vi "configuration UI.vi"() -> ()   [LabVIEW 2013, in "Shared Library Module editor node.lvclass"]
doc: "Platypus Framework 1.0.1.60\nNI Systems Engineering - National Instruments"
uses:
  Shared Library Module editor node.lvclass
  <vilib>/NI/Configuration Framework/Node/NodeRef.ctl
  <vilib>/NI/Configuration Framework/Node/NISE_CEF_Node.lvclass
  <vilib>/NI/AMC/Message Queue.ctl
  <vilib>/NI/AMC/Message.ctl
  <vilib>/NI/Tools/Keyed Array/KeyedArray.ctl
  <vilib>/NI/Configuration Framework/Node/UserEventRef.ctl
  <vilib>/NI/Configuration Framework/Controls/EventCluster.ctl
  <vilib>/NI/DCAF UI Toolkit/Controls/Configure.ctl
  <vilib>/NI/DCAF UI Toolkit/Controls/Add.ctl
  <vilib>/NI/DCAF UI Toolkit/Controls/Remove.ctl
  <vilib>/NI/DCAF UI Toolkit/Controls/Import.ctl
  configuration/Shared Library Module configuration.lvclass
  <vilib>/Utility/miscctls.llb/LVPositionTypeDef.ctl
  <vilib>/NI/Module Execution Interface/Engine Configuration/engine configuration.lvclass
  <vilib>/NI/Tag Bus Data Framework/Configuration Editor/Classes/Engine Parent/Engine Parent Editor Node.lvclass
  <vilib>/NI/Configuration Framework/serializable configuration/NISE_CEF_serializable configuration.lvclass/NISE_CEF_serializable configuration.ctl
  configuration/Shared Library Module configuration.lvclass/Shared Library Module configuration.ctl
  <vilib>/NI/Tag Bus/tag/tag descriptor.lvclass/tag descriptor.ctl
  <vilib>/NI/Tag Bus/tag/write tag name.vi
  configuration/Write args.vi
  configuration/Write dllpath.vi
  Write local path.vi
  Read local path.vi
  <vilib>/NI/Configuration Framework/serializable configuration/Read UID.vi
  configuration/Read args.vi
  configuration/Read dllpath.vi
  <vilib>/NI/Tag Bus Data Framework/Configuration Editor/Classes/Module editor node/Read Module Configuration.vi
  <vilib>/NI/Configuration Framework/serializable configuration/read metadata property.vi
  <vilib>/NI/Tag Bus Data Framework/Configuration Editor/Classes/Module editor node/Write Module Configuration.vi
  <vilib>/Utility/LVClass/Get LV Class Name.vi
  <vilib>/NI/Configuration Framework/error generator/NISE_error generator.vi
  <vilib>/NI/Configuration Framework/serializable configuration/set metadata property.vi
  <vilib>/NI/Configuration Framework/serializable configuration/NISE_CEF_serializable configuration.lvclass
  <vilib>/NI/Tag Bus Module Framework/module configuration/TBM module configuration.lvclass
  <vilib>/NI/Configuration Framework/NISE_CEF_TreeControl.lvlib
  <vilib>/NI/Tag Bus Data Framework/Configuration Editor/Classes/Module editor node/module editor node.lvclass
  <vilib>/NI/Tag Bus Module Framework/channel/TBM channel.lvclass
  <vilib>/NI/Tools/Keyed Array/Tools_KeyedArray.lvlib
  <vilib>/NI/AMC/AMC.lvlib
  <vilib>/NI/DCAF UI Toolkit/Controls/DCAF UI Elements.lvlib
panel:
  in  "Top Level Tab Control":T1(tab)
  in  "Open Button":T2
  in  "settings":T3
  in  "channel":i32(listbox)
  in  "Add Button":T4
  in  "Remove Button":T5
  in  "Additional Arguments":string[](array[string])
  in  "Library Path (required)":path
  in  "Local Library Path (optional)":path
  in  "user event":T6
  in  "main queue":T7
  in  "node ref":T8
  # "It is recommended that libraries are placed in the default search path. For example, on Linux RT this would be /usr/lib, while VxWorks places it at /ni-rt/system.\n\nIf this is the case, libraries can be referenced by name. To make the name cross-platform, wildcards can be specified.\n\nLibname.* becomes libname.dll on windows and libname.so on Linux.\n\nLibname*.* becomes Libname32.* on 32-bit operating systems/environments and Libname64.* on 64-bit operating systems/environments."
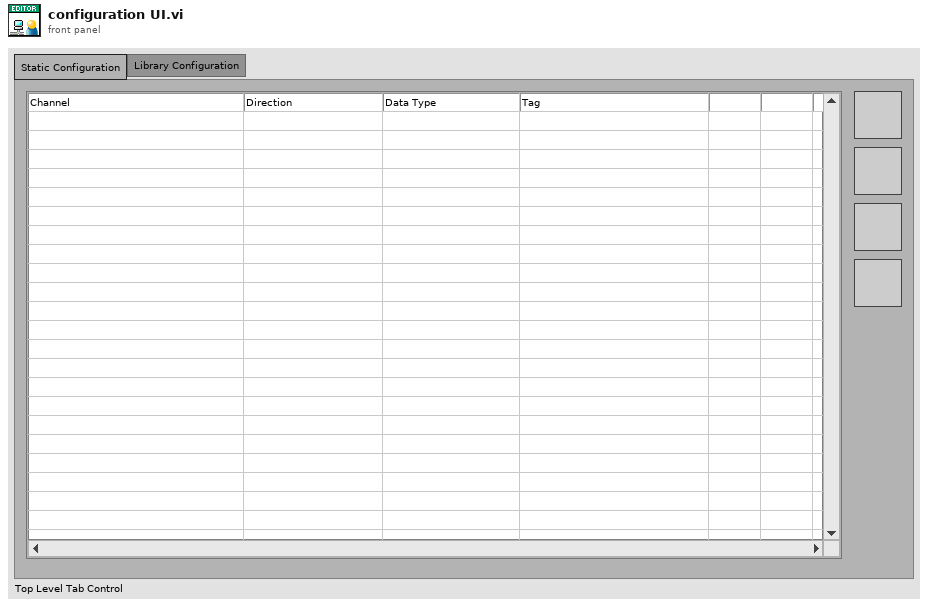
[diagram p1: front panel]
types:
  T1 = enum32{"Static Configuration", "Library Configuration"}
  T2 = typedef "DCAF UI Elements.lvlib/Import.ctl" = bool
  T3 = typedef "DCAF UI Elements.lvlib/Configure.ctl" = bool
  T4 = typedef "DCAF UI Elements.lvlib/Add.ctl" = bool
  T5 = typedef "DCAF UI Elements.lvlib/Remove.ctl" = bool
  T6 = typedef "NISE_CEF_Node.lvclass/UserEventRef.ctl" = refnum<user-event>
  T7 = typedef "AMC.lvlib/Message Queue.ctl" = refnum<queue>
  T8 = typedef "NISE_CEF_Node.lvclass/NodeRef.ctl" = refnum<data-value>
  T9 = typedef "LVPositionTypeDef.ctl" = cluster{"Left":i32, "Top":i32}
  T10 = typedef "NISE_CEF_TreeControl.lvlib/EventCluster.ctl" = cluster{"command":string, "data":string}
  T11 = typedef "Shared Library Module editor node.lvclass/table line.ctl" = cluster{"channel in":refnum<class "TBM channel.lvclass">, "tag name":string}
  T12 = typedef "TBM channel.lvclass/channel classification.ctl" = enum16{"input data", "output data", "processing parameter", "processing result"}
  T13 = typedef "tag bus.lvlib/tag descriptor.lvclass/Data Type.ctl" = enum16{"Double", "Single", "I64", "I32", "I16", "I8", "U64", "U32", "U16", "U8", "Boolean", "String", "Array of Double", "Array of Single", "Array of I64", "Array of I32", "Array of I16", "Array of I8", "Array of U64", "Array of U32", "Array of U16", "Array of U8", "Array of Boolean", "Array of String"}
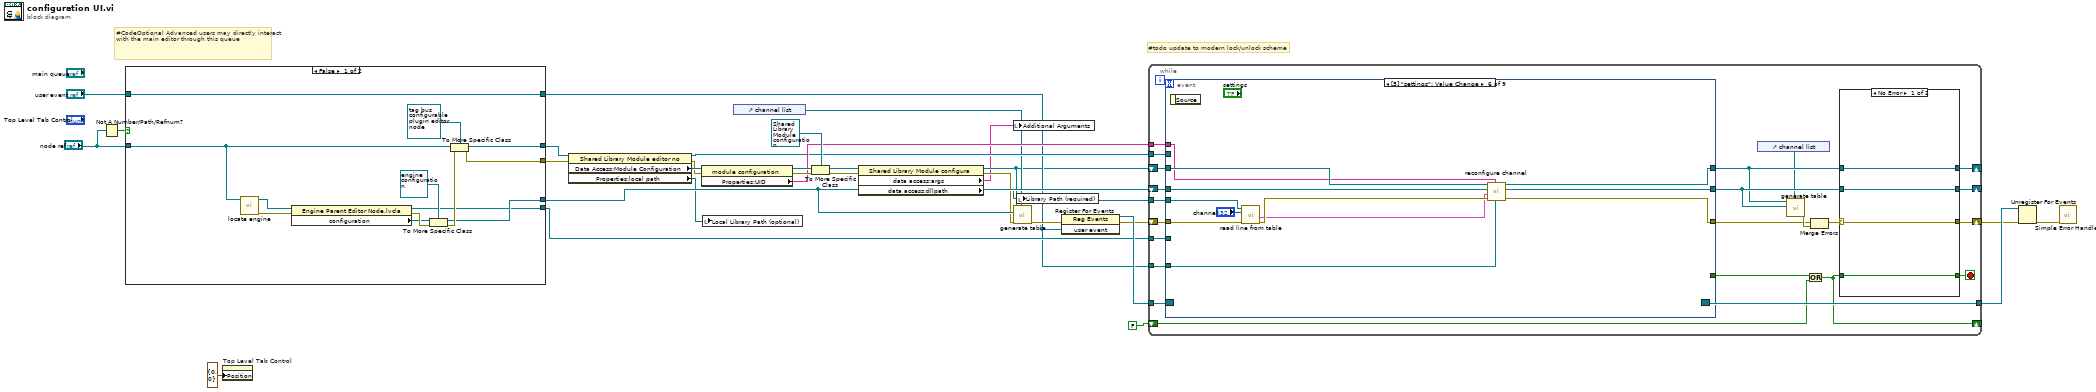
[diagram p0: block diagram]
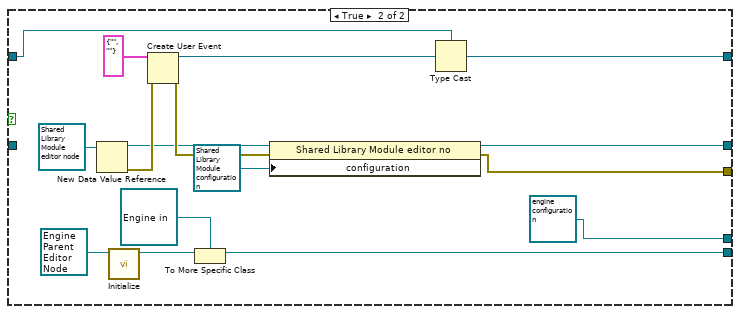
[diagram p2: hidden frame]
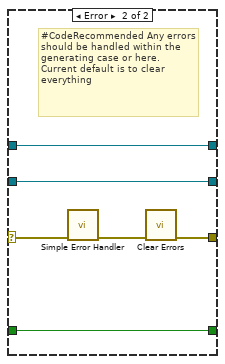
[diagram p3: hidden frame]
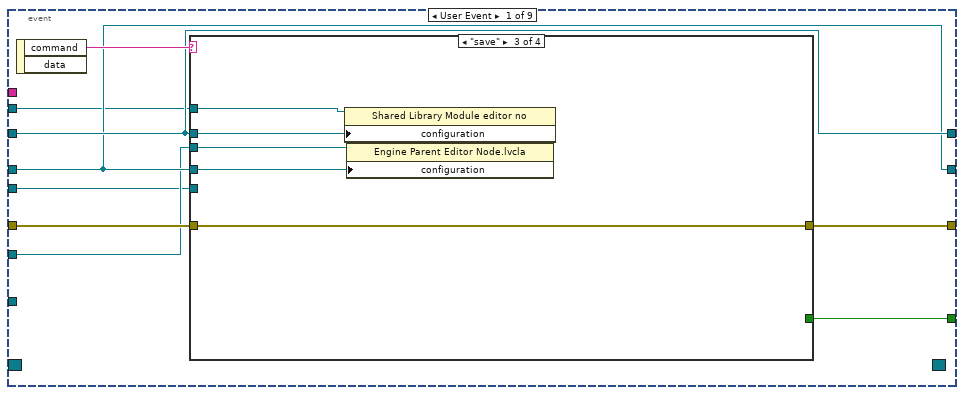
[diagram p4: hidden frame]
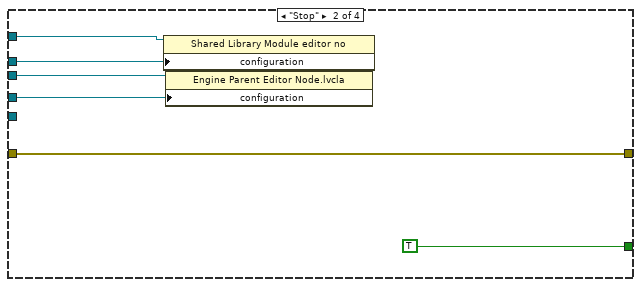
[diagram p6: hidden frame]
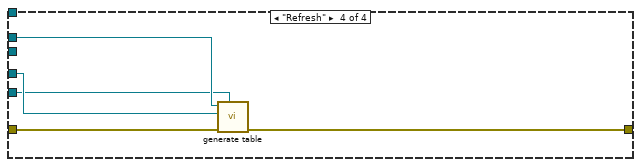
[diagram p7: hidden frame]
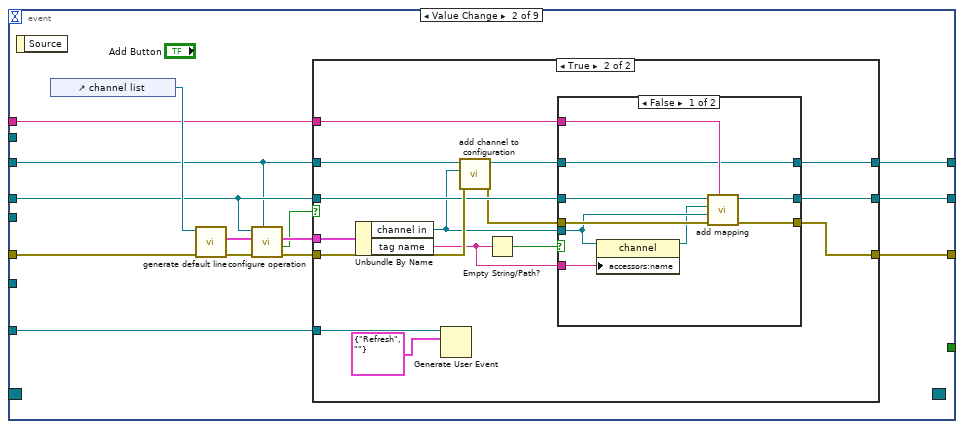
[diagram p8: hidden frame]
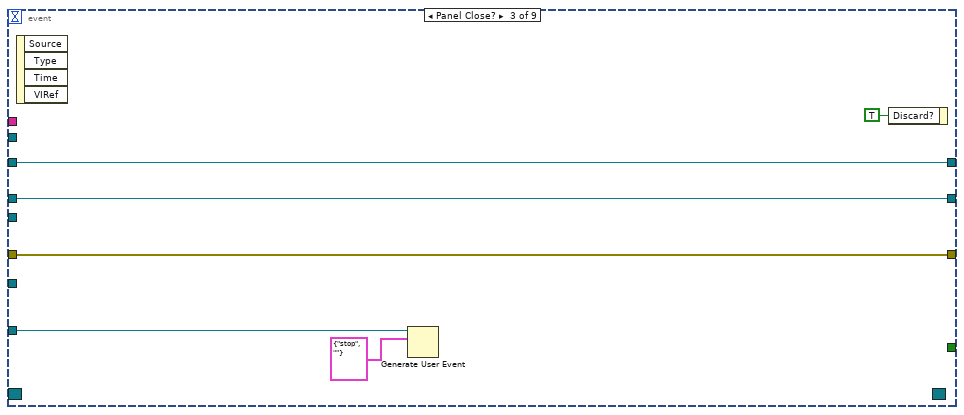
[diagram p11: hidden frame]
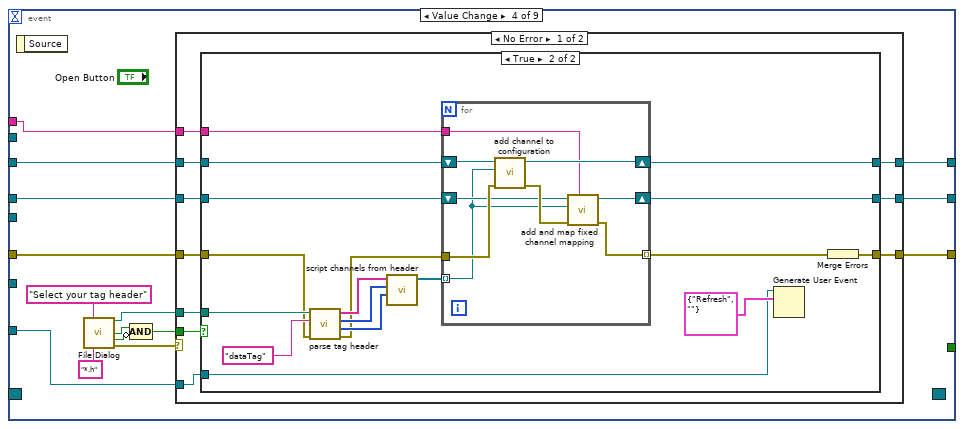
[diagram p12: hidden frame]
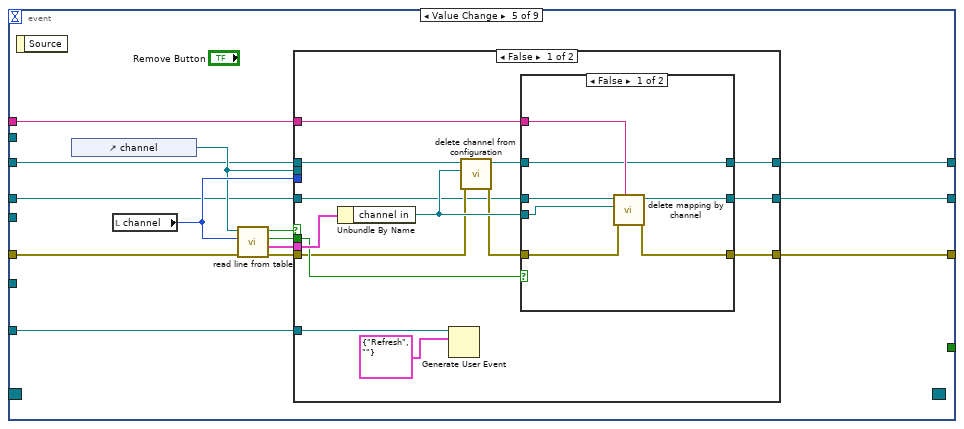
[diagram p15: hidden frame]
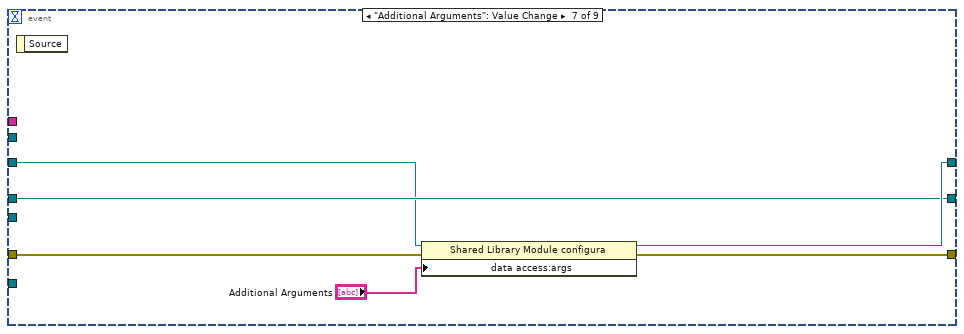
[diagram p18: hidden frame]
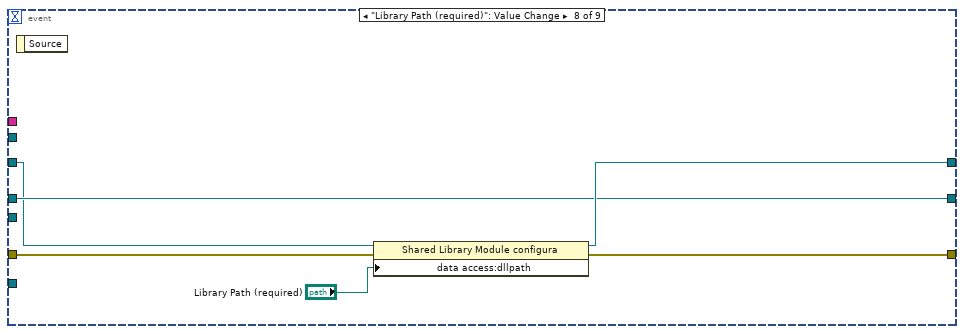
[diagram p19: hidden frame]
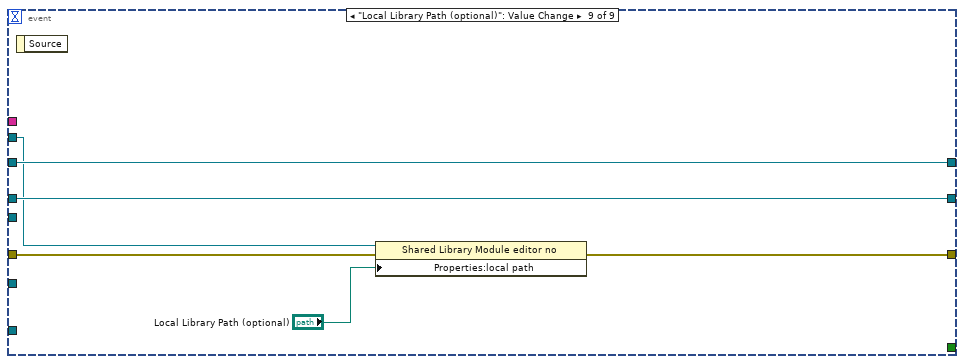
[diagram p20: hidden frame]
diagram:
  # "#todo update to modern lock/unlock scheme"
  # "#CodeOptional Advanced users may directly interact with the main editor through this queue"
  n1 = Not A Number/Path/Refnum?(number/path/refnum="node ref") -> (NaN/Path/Refnum?=w22:bool)
  n2 = case shown="False" w22 {
    tunnel: "user event" -> [w44 w46]
    tunnel: [w44 w47] -> w8
    tunnel: "node ref" -> [w42 _]
    tunnel: [w41 w54] -> w15
    tunnel: [w40 w48] -> w20
    tunnel: [w33 refnum<class "engine configuration.lvclass"> refnum ("Engine Configuration")] -> w17
    tunnel: [w32 w51] -> w11
    frame False {
      n3 = call <vilib>:"locate engine.vi"("component"=w42) -> ("error out"=w37:errorcluster, "engine"=w39:refnum<data-value>)  [unwired: 9 in]
      n4 = property class="Engine Parent Editor Node.lvcla"(reference=w39, error in=w37) -> (reference out=w32:refnum<data-value>, error out=w36:errorcluster, "configuration"=w35:refnum<class "NISE_CEF_serializable configuration.lvclass">)
      n5 = To More Specific Class(target class=refnum<class "engine configuration.lvclass"> refnum ("engine configuration.lvclass"), reference=w35, error in=w36) -> (specific class reference=w33:refnum<class "engine configuration.lvclass">, error out=w34:errorcluster)
      n6 = To More Specific Class(target class=refnum<data-value> refnum ("data value reference"), reference=w42, error in=w34) -> (specific class reference=w41:refnum<data-value>, error out=w40:errorcluster)
    }
    frame True {
      n7 = New Data Value Reference(data value=refnum<class "Shared Library Module editor node.lvclass"> refnum ("tag bus configurable plugin editor node")) -> (data value reference=w53:refnum<data-value>, error out=w56:errorcluster)  [unwired: 1 in]
      n8 = call-dynamic "Initialize.vi"("Engine in"=refnum<class "Engine Parent Editor Node.lvclass"> refnum) -> ("data value reference"=w52:T8)  [unwired: 8 in, 2 out]
      n9 = Create User Event(user event datatype=T10 {"command"="", "data"=""} ("event data"), error in=w56) -> (user event=w59:refnum<user-event>, error out=w55:errorcluster)
      n10 = To More Specific Class(target class=refnum<data-value> refnum ("data value reference"), reference=w52) -> (specific class reference=w51:refnum<data-value>)  [unwired: 1 in, 1 out]
      n11 = property class="Shared Library Module editor no"(reference=w53, error in=w55, "configuration"=refnum<class "Shared Library Module configuration.lvclass"> refnum ("tag bus configurable plugin module configuration")) -> (reference out=w54:refnum<data-value>, error out=w48:errorcluster)
      n12 = Type Cast(type=w46, x=w59) -> (*(type *) &x=w47:T6)
    }
  }
  n13 = property on="Top Level Tab Control" class="TabCtl (strict)"("Position"=T9 {"Left"=0, "Top"=0}) -> ()  [unwired: 2 in, 2 out]
  n14 = property class="Shared Library Module editor no"(reference=w15, error in=w20) -> (reference out=w10:refnum<data-value>, error out=w25:errorcluster, "Data Access:Module Configuration"=w26:refnum<class "TBM module configuration.lvclass">, "Properties:local path"=w7:path)
  n15 = property class="module configuration"(reference=w26, error in=w25) -> (reference out=w23:refnum<class "TBM module configuration.lvclass">, error out=w24:errorcluster, "Properties:UID"=w19:string)
  n16 = local write "Local Library Path (optional)"(w7) -> ()
  n17 = control-ref of="channel list"() -> (w9:refnum<vi>)
  n18 = To More Specific Class(target class=refnum<class "Shared Library Module configuration.lvclass"> refnum ("tag bus configurable plugin module configuration"), reference=w23, error in=w24) -> (specific class reference=w5:refnum<class "Shared Library Module configuration.lvclass">, error out=w16:errorcluster)
  n19 = property class="Shared Library Module configura"(reference=w5, error in=w16) -> (reference out=w4:refnum<class "Shared Library Module configuration.lvclass">, error out=w6:errorcluster, "data access:args"=w2:string[], "data access:dllpath"=w3:path)
  n20 = local write "Additional Arguments"(w2) -> ()
  n21 = call "generate table.vi"("table"=w9, "error in"=w6, "engine configuration in"=w17, "Shared Library Module configuration in"=w4) -> ("error out"=w14:errorcluster)  [unwired: 7 in]
  n22 = local write "Library Path (required)"(w3) -> ()
  n23 = register-events(error in=w14, w8) -> (reference out=w31:refnum<event-registration>, error out=w13:errorcluster)  [unwired: 1 in]
  n24 = while {
    tunnel: w31 -> [w83]
    tunnel: [w82] -> w30
    shift-right: [w76] -> w29
    shift-left: w13 -> [w81]
    shift-right: [w78] -> _
    shift-left: FALSE -> [w77]
    shift-right: [w72] -> _
    shift-left: w4 -> [w75]
    shift-right: [w73] -> _
    shift-left: w17 -> [w74]
    tunnel: w19 -> [w71]
    tunnel: w11 -> [w64]
    tunnel: w10 -> [w63]
    tunnel: w9 -> [w62]
    tunnel: w8 -> [w61]
    stop <- w80 stop-if-true
    n25 = event shown="[5] \"settings\": Value Change" {
      selector: w83 -> [_ _ _ _ _ _ _ _ _]
      dyn-events: [_ _ _ _ _ _ _ _ _] -> w82
      timeout: _ -> [_ _ _ _ _ _ _ _ _]
      tunnel: [w102 _ _ _ _ _ _ _ _] -> w79
      tunnel: [w100 w133 w169 w178 w240 w278 w284 w290 w294] -> w66
      tunnel: w81 -> [w99 w132 w169 w177 w239 w279 w285 w291 w297]
      tunnel: w75 -> [w98 w121 w167 w174 w235 w274 w280 w286 w295]
      tunnel: w74 -> [w97 w122 w166 w175 w234 w275 w281 w287 w296]
      tunnel: [w97 w126 w166 w176 w229 w272 w281 w287 w296] -> w70
      tunnel: [w98 w125 w167 w173 w228 w273 w283 w289 w295] -> w69
      tunnel: w71 -> [_ w124 _ w171 w230 w270 _ _ _]
      tunnel: w64 -> [w96 _ _ _ _ _ _ _ _]
      tunnel: w63 -> [w95 _ _ _ _ _ _ _ w293]
      tunnel: w62 -> [w94 _ _ _ _ w271 _ _ _]
      tunnel: w61 -> [_ w120 w165 w170 w227 w268 _ _ _]
      event User Event {
        n26 = event-data() -> ("command"=w101:string)  [unwired: 1 in, 1 out]
        n27 = case shown="\"save\"" w101 {
          tunnel: [_ TRUE _ _] -> w102
          tunnel: [w103 w108 w114 w116] -> w100
          tunnel: w99 -> [w103 w108 w114 w119]
          tunnel: w98 -> [_ w107 w113 w118]
          tunnel: w97 -> [_ w106 w112 w117]
          tunnel: w96 -> [_ w105 w111 _]
          tunnel: w95 -> [_ w104 w110 _]
          tunnel: w94 -> [_ _ _ w115]
          frame Default {
          }
          frame "Stop" {
            n28 = property class="Shared Library Module editor no"(reference=w104, "configuration"=w107) -> ()  [unwired: 1 in, 2 out]
            n29 = property class="Engine Parent Editor Node.lvcla"(reference=w105, "configuration"=w106) -> ()  [unwired: 1 in, 2 out]
          }
          frame "save" {
            n30 = property class="Shared Library Module editor no"(reference=w110, "configuration"=w113) -> ()  [unwired: 1 in, 2 out]
            n31 = property class="Engine Parent Editor Node.lvcla"(reference=w111, "configuration"=w112) -> ()  [unwired: 1 in, 2 out]
          }
          frame "Refresh" {
            n32 = call "generate table.vi"("table"=w115, "error in"=w119, "engine configuration in"=w117, "Shared Library Module configuration in"=w118) -> ("error out"=w116:errorcluster)  [unwired: 7 in]
          }
        }
      }
      event Value Change {
        n33 = event-data() -> ()  [unwired: 1 in, 1 out]
        n34 = control-ref of="channel list"() -> (w131:refnum<vi>)
        n35 = call "generate default line.vi"("error in"=w132, "operations table"=w131) -> ("error out"=w129:errorcluster, "line"=w130:T11)  [unwired: 8 in]
        n36 = call "configure operation.vi"("Shared Library Module configuration in"=w121, "error in"=w129, "line item in"=w130, "engine configuration in"=w122) -> ("error out"=w127:errorcluster, "success"=w123:bool, "line item out"=w128:T11)  [unwired: 4 in, 1 out]
        n37 = case shown="True" w123 {
          tunnel: [w136 w139] -> w133
          tunnel: w127 -> [w136 w149]
          tunnel: w122 -> [w135 w147]
          tunnel: w128 -> [_ w150]
          tunnel: w121 -> [w134 w151]
          tunnel: [w135 w146] -> w126
          tunnel: [w134 w140] -> w125
          tunnel: w124 -> [_ w143]
          tunnel: w120 -> [_ w137]
          frame False {
          }
          frame True {
            n38 = Unbundle By Name(w150) -> ("channel in"=w144:refnum<class "TBM channel.lvclass">, "tag name"=w142:string)
            n39 = Generate User Event(user event=w137, event data cluster=T10 {"command"="Refresh", "data"=""} ("event data")) -> ()  [unwired: 2 in, 2 out]
            n40 = call "add channel to configuration.vi"("error in"=w149, "TBM channel in"=w144, "Shared Library Module configuration in"=w151) -> ("error out"=w145:errorcluster, "Shared Library Module configuration out"=w141:refnum<class "Shared Library Module configuration.lvclass">)  [unwired: 7 in]
            n41 = Empty String/Path?(string/path=w142) -> (empty?=w148:bool)
            n42 = case shown="False" w148 {
              tunnel: w147 -> [w160 w163]
              tunnel: [w159 w163] -> w146
              tunnel: w145 -> [w158 w162]
              tunnel: w144 -> [w156 _]
              tunnel: w143 -> [w157 _]
              tunnel: w142 -> [w155 _]
              tunnel: [w153 w162] -> w139
              tunnel: w141 -> [w152 w161]
              tunnel: [w152 w161] -> w140
              frame False {
                n43 = property class="channel"(reference=w156, "accessors:name"=w155) -> (reference out=w154:refnum<class "TBM channel.lvclass">)  [unwired: 1 in, 1 out]
                n44 = call <vilib>:"add mapping.vi"("owner ID"=w157, "error in"=w158, "channel"=w156, "tag descriptor"=w154, "engine configuration"=w160) -> ("error out"=w153:errorcluster, "engine configuration out"=w159:refnum<class "engine configuration.lvclass">)  [unwired: 5 in]
              }
              frame True {
              }
            }
          }
        }
      }
      event Panel Close? {
        n45 = event-data() -> ()  [unwired: 1 in, 4 out]
        n46 = Generate User Event(user event=w165, event data cluster=T10 {"command"="stop", "data"=""} ("event data")) -> ()  [unwired: 2 in, 2 out]
        n47 = event-data("Discard?"=TRUE) -> ()  [unwired: 1 in, 1 out]
      }
      event Value Change {
        n48 = event-data() -> ()  [unwired: 1 in, 1 out]
        n49 = call "File Dialog"("prompt"="Select your tag header", "pattern (all files)"="*.h") -> ("selected path"=w172:path, "exists"=w181:bool, "cancelled"=w180:bool, "error out"=w182:errorcluster)  [unwired: 10 in]
        n50 = Compound Arithmetic op=AND(w181, invert w180) -> (w179:bool)
        n51 = case shown="No Error" w182 {
          tunnel: w179 -> [w194 _]
          tunnel: [w193 w226] -> w178
          tunnel: w177 -> [w192 w226]
          tunnel: [w190 w225] -> w176
          tunnel: w175 -> [w191 w225]
          tunnel: w174 -> [w188 w224]
          tunnel: [w189 w224] -> w173
          tunnel: w172 -> [w187 _]
          tunnel: w171 -> [w186 _]
          tunnel: w170 -> [w185 _]
          frame No Error {
            n52 = case shown="True" w194 {
              tunnel: [w197 w203] -> w193
              tunnel: w192 -> [w197 w209]
              tunnel: w191 -> [w196 w207]
              tunnel: [w196 w206] -> w190
              tunnel: [w195 w205] -> w189
              tunnel: w188 -> [w195 w208]
              tunnel: w187 -> [_ w210]
              tunnel: w186 -> [_ w200]
              tunnel: w185 -> [_ w198]
              frame False {
              }
              frame True {
                n53 = call "parse tag header.vi"("error in"=w209, "tag type name"="dataTag", "Path"=w210) -> ("error out"=w204:errorcluster, "classifications"=w214:T12[], "types"=w213:T13[], "names"=w212:string[])  [unwired: 5 in]
                n54 = call "script channels from header.vi"("classifications"=w214, "types"=w213, "names"=w212) -> ("channels"=w202:refnum<class "TBM channel.lvclass">[])  [unwired: 8 in]
                n55 = for {
                  shift-right: [w216] -> w205
                  shift-left: w208 -> [w223]
                  shift-right: [w217] -> w206
                  shift-left: w207 -> [w219]
                  tunnel: w204 -> [w222]
                  tunnel: w202 -> [w218] mode=indexing
                  tunnel: [w220] -> w201 mode=indexing
                  tunnel: w200 -> [w215]
                  n56 = call "add channel to configuration.vi"("error in"=w222, "TBM channel in"=w218, "Shared Library Module configuration in"=w223) -> ("error out"=w221:errorcluster, "Shared Library Module configuration out"=w216:refnum<class "Shared Library Module configuration.lvclass">)  [unwired: 7 in]
                  n57 = call <vilib>:"add and map fixed channel mapping.vi"("module instance"=w215, "error in"=w221, "fixed channel"=w218, "engine configuration in"=w219) -> ("error out"=w220:errorcluster, "engine configuration out"=w217:refnum<class "engine configuration.lvclass">)  [unwired: 6 in]
                }
                n58 = Generate User Event(user event=w198, event data cluster=T10 {"command"="Refresh", "data"=""} ("event data")) -> ()  [unwired: 2 in, 2 out]
                n59 = Merge Errors(w201) -> (w203:errorcluster)
              }
            }
          }
          frame Error {
          }
        }
      }
      event Value Change {
        n60 = event-data() -> ()  [unwired: 1 in, 1 out]
        n61 = control-ref of="channel"() -> (w237:refnum<vi>)
        n62 = local read "channel"() -> (w238:i32)
        n63 = call "read line from table.vi"("error in"=w239, "line number"=w238, "operations table"=w237) -> ("error out"=w231:errorcluster, "line"=w236:T11, "empty tag?"=w232:bool, "empty channel?"=w233:bool)  [unwired: 5 in]
        n64 = case shown="False" w233 {
          tunnel: [w243 w266] -> w240
          tunnel: w238 -> [_ _]
          tunnel: w237 -> [_ _]
          tunnel: w236 -> [w254 _]
          tunnel: w235 -> [w252 w265]
          tunnel: w234 -> [w247 w267]
          tunnel: w232 -> [w253 _]
          tunnel: w231 -> [w250 w266]
          tunnel: w230 -> [w246 _]
          tunnel: [w245 w267] -> w229
          tunnel: [w244 w265] -> w228
          tunnel: w227 -> [w241 _]
          frame False {
            n65 = Unbundle By Name(w254) -> ("channel in"=w251:refnum<class "TBM channel.lvclass">)
            n66 = Generate User Event(user event=w241, event data cluster=T10 {"command"="Refresh", "data"=""} ("event data")) -> ()  [unwired: 2 in, 2 out]
            n67 = call "delete channel from configuration.vi"("error in"=w250, "TBM channel in"=w251, "Shared Library Module configuration in"=w252) -> ("error out"=w248:errorcluster, "Shared Library Module configuration out"=w249:refnum<class "Shared Library Module configuration.lvclass">)  [unwired: 7 in]
            n68 = case shown="False" w253 {
              tunnel: w251 -> [w260 _]
              tunnel: w249 -> [w255 w262]
              tunnel: w248 -> [w258 w263]
              tunnel: w247 -> [w261 w264]
              tunnel: w246 -> [w259 _]
              tunnel: [w257 w264] -> w245
              tunnel: [w256 w263] -> w243
              tunnel: [w255 w262] -> w244
              frame False {
                n69 = call <vilib>:"delete mapping by channel.vi"("owner ID"=w259, "error in"=w258, "channel"=w260, "engine configuration in"=w261) -> ("error out"=w256:errorcluster, "engine configuration out"=w257:refnum<class "engine configuration.lvclass">)  [unwired: 6 in]
              }
              frame True {
              }
            }
          }
          frame True {
          }
        }
      }
      event Value Change {
        n70 = event-data() -> ()  [unwired: 1 in, 1 out]
        n71 = call "read line from table.vi"("error in"=w279, "line number"="channel", "operations table"=w271) -> ("error out"=w277:errorcluster, "line"=w269:T11)  [unwired: 5 in, 2 out]
        n72 = call "reconfigure channel.vi"("user event"=w268, "instance identifier"=w270, "error in"=w277, "line"=w269, "Data Access:Engine Configuration"=w275, "Shared Library Module configuration in"=w274) -> ("error out"=w278:errorcluster, "engine configuration out"=w272:refnum<class "engine configuration.lvclass">, "Shared Library Module configuration out"=w273:refnum<class "Shared Library Module configuration.lvclass">)  [unwired: 3 in]
      }
      event "Additional Arguments": Value Change {
        n73 = event-data() -> ()  [unwired: 1 in, 1 out]
        n74 = property class="Shared Library Module configura"(reference=w280, error in=w285, "data access:args"="Additional Arguments") -> (reference out=w283:refnum<class "Shared Library Module configuration.lvclass">, error out=w284:errorcluster)
      }
      event "Library Path (required)": Value Change {
        n75 = event-data() -> ()  [unwired: 1 in, 1 out]
        n76 = property class="Shared Library Module configura"(reference=w286, error in=w291, "data access:dllpath"="Library Path (required)") -> (reference out=w289:refnum<class "Shared Library Module configuration.lvclass">, error out=w290:errorcluster)
      }
      event "Local Library Path (optional)": Value Change {
        n77 = event-data() -> ()  [unwired: 1 in, 1 out]
        n78 = property class="Shared Library Module editor no"(reference=w293, error in=w297, "Properties:local path"="Local Library Path (optional)") -> (error out=w294:errorcluster)  [unwired: 1 out]
      }
    }
    n79 = control-ref of="channel list"() -> (w68:refnum<vi>)
    n80 = call "generate table.vi"("table"=w68, "engine configuration in"=w70, "Shared Library Module configuration in"=w69) -> ("error out"=w67:errorcluster)  [unwired: 8 in]
    n81 = Or(x=w79, y=w77) -> (x .or. y?=w78:bool)
    n82 = Merge Errors(w66, w67) -> (w65:errorcluster)
    n83 = case shown="No Error" w65 {
      selector: w65 -> [w84 w92]
      tunnel: [w87 w93] -> w80
      tunnel: w78 -> [w87 w93]
      tunnel: [w84 w90] -> w76
      tunnel: w70 -> [w85 w89]
      tunnel: [w85 w89] -> w73
      tunnel: w69 -> [w86 w88]
      tunnel: [w86 w88] -> w72
      frame No Error {
      }
      frame Error {
        # "#CodeRecommended Any errors should be handled within the generating case or here. Current default is to clear everything"
        n84 = call <vilib>:"Simple Error Handler.vi"("error in (no error)"=w92) -> ("error out"=w91:errorcluster)  [unwired: 4 in, 4 out]
        n85 = call <vilib>:"Clear Errors.vi"("error in (no error)"=w91) -> ("error out"=w90:errorcluster)  [unwired: 6 in]
      }
    }
  }
  n86 = Unregister For Events(event registration refnum=w30, error in=w29) -> (error out=w12:errorcluster)
  n87 = call <vilib>:"Simple Error Handler.vi"("error in (no error)"=w12) -> ()  [unwired: 4 in, 5 out]
